vi "MsgCF.vi"(8 "error in":errorcluster, 11 "DataIn":u8[](array[numeric]) format="%02x") -> (0 "error out":errorcluster, 2 "SN":i32, 3 "CF Data Bytes":u8[](array[numeric]) format="%02x")   [LabVIEW 2011, in "Konvolucio MUDS150628.lvlib"]
uses:
  <instrlib>/Konvolucio MUDS150628/Konvolucio MUDS150628.lvlib
panel:
  out "x << y":u8
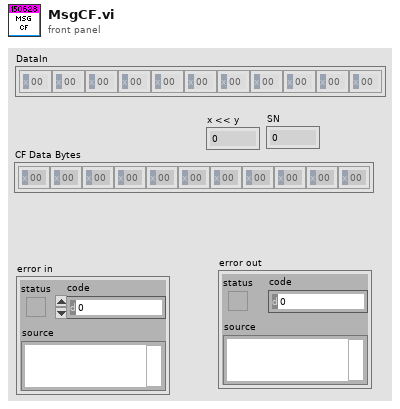
[diagram p1: front panel]
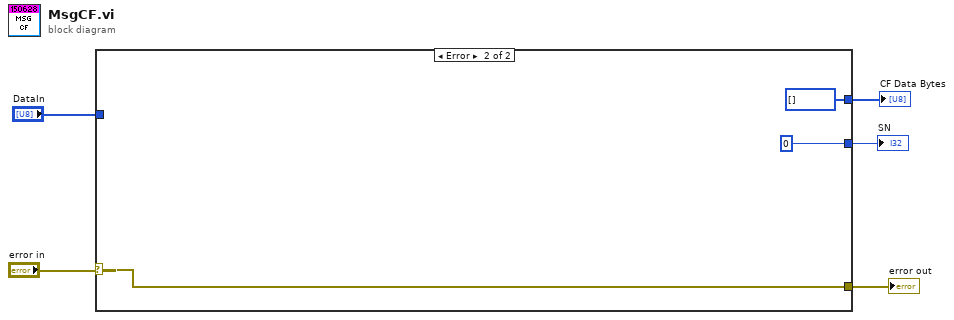
[diagram p0: block diagram]
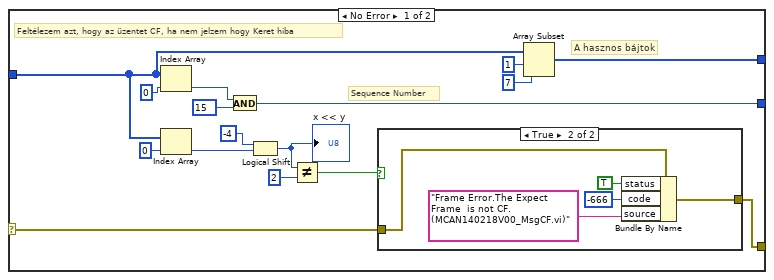
[diagram p2: hidden frame]
diagram:
  n1 = case shown="Error" "error in" {
    selector: "error in" -> [w11 w30]
    tunnel: [w10 w30] -> w5
    tunnel: [w17 0] -> w3
    tunnel: [w7 u8[] []] -> w2
    tunnel: "DataIn" -> [w6 _]
    frame No Error {
      # "A hasznos bájtok"
      # "Sequence Number"
      # "Feltélezem azt, hogy az üzentet CF, ha nem jelzem hogy Keret hiba"
      n2 = Index Array(array=w6, index=0) -> (element=w20:u8)
      n3 = Index Array(array=w6, index=0) -> (element=w15:u8)
      n4 = And(x=w20, y=u8 15) -> (x .and. y?=w17:u8)
      n5 = Logical Shift(y=i8 -4, x=w15) -> (x << y=w14:u8)
      "x << y" <- w14
      n6 = Not Equal?(x=w14, y=u8 2) -> (x != y?=w12:bool)
      n7 = case shown="True" w12 {
        tunnel: w11 -> [w22 w27]
        tunnel: [w22 w23] -> w10
        frame False {
        }
        frame True {
          n8 = Bundle By Name(cluster=w27, "status"=TRUE, "code"=-666, "source"="Frame Error.The Expect Frame  is not CF. (MCAN140218V00_MsgCF.vi)") -> (w23:errorcluster)
        }
      }
      n9 = Array Subset(array=w6, index=1, length=7) -> (w7:u8[])
    }
    frame Error {
    }
  }
  "error out" <- w5
  "SN" <- w3
  "CF Data Bytes" <- w2
